vi "Write Timing Status.vi"(8 "error in":errorcluster, 11 "framework performance in":refnum<class "Performance.lvclass">) -> (0 "error out":errorcluster, 3 "framework performance out":refnum<class "Performance.lvclass">)   [LabVIEW 2017, in "DSF Core.lvlib" / "Performance.lvclass"]
uses:
  Performance.lvclass
  Performance.lvclass/Performance.ctl
  Timing Status/Timing Status Pointer.lvclass
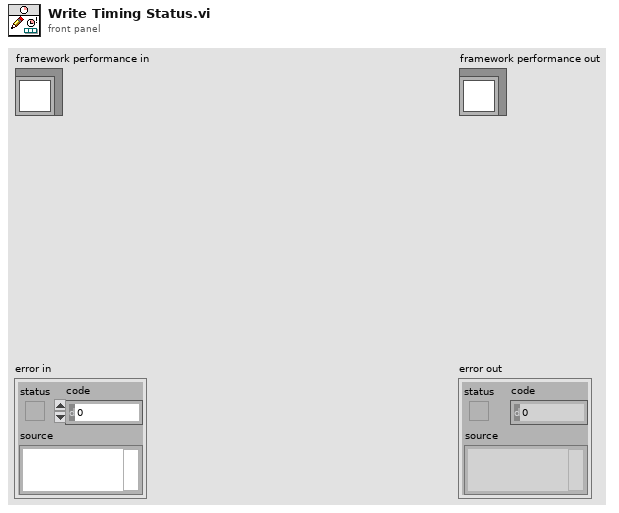
[diagram p1: front panel]
types:
  T1 = typedef "DSF Core.lvlib/Timing Status Pointer.lvclass/Timing Status Data.ctl" = cluster{"rx start time":u32, "rx end time":u32, "tx start time":u32, "tx end time":u32, "cycle start time":u32, "cycle end time":u32, "prev start time":u32}
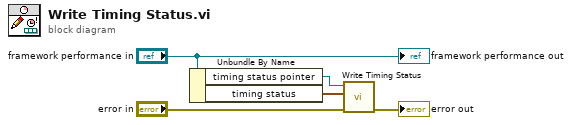
[diagram p0: block diagram]
diagram:
  n1 = Unbundle By Name("framework performance in") -> ("timing status pointer"=w5:refnum<class "Timing Status Pointer.lvclass">, "timing status"=w1:T1)
  n2 = call "Write Timing Status.vi"("error in (no error)"="error in", "timing status"=w1, "timing status pointer in"=w5) -> ("error out"=→"error out":errorcluster)  [unwired: 7 in, 1 out]
  "framework performance out" <- "framework performance in"
